vi "GetControlRefsFromVi.vi"(11 "VI Refnum":refnum<vi>) -> (0 "error out":errorcluster, 3 "Variant":variant)   [LabVIEW 2016, in "M1M3SupportEUI_Views.lvlib"]
uses:
  M1M3SupportEUI_Views.lvlib
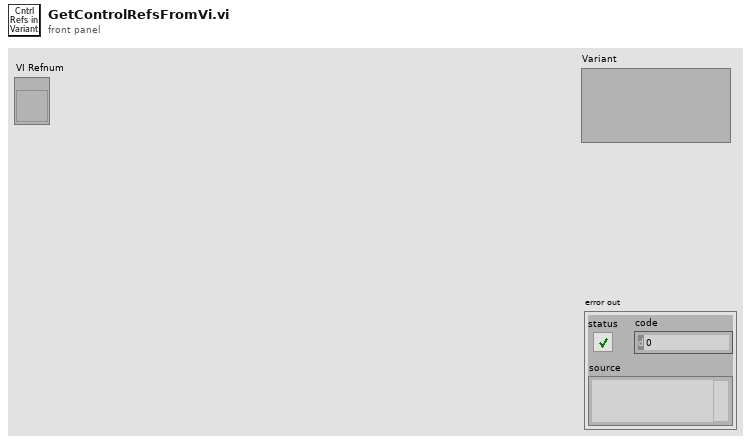
[diagram p1: front panel]
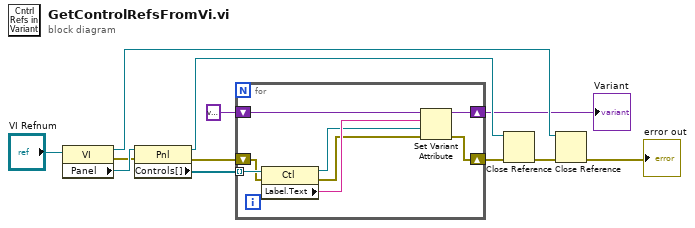
[diagram p0: block diagram]
diagram:
  n1 = property class="VI"(reference="VI Refnum") -> (reference out=w12:refnum<vi>, error out=w4:errorcluster, "Panel"=w5:refnum<vi>)  [unwired: 1 in]
  n2 = property class="Pnl"(reference=w5, error in=w4) -> (reference out=w11:refnum<vi>, error out=w8:errorcluster, "Controls[]"=w6:refnum<vi>[])
  n3 = for {
    tunnel: w6 -> [w20] mode=indexing
    shift-right: [w16] -> w2
    shift-left: variant -> [w19]
    shift-right: [w13] -> w10
    shift-left: w8 -> [w15]
    n4 = property class="Ctl"(reference=w20, error in=w15) -> (reference out=w17:refnum<vi>, error out=w14:errorcluster, "Label.Text"=w18:string)
    n5 = Set Variant Attribute(Variant=w19, name=w18, value=w17, error in=w14) -> (Variant out=w16:variant, error out=w13:errorcluster)  [unwired: 1 out]
  }
  "Variant" <- w2
  n6 = Close Reference(reference=w11, error in (no error)=w10) -> (error out=w9:errorcluster)
  n7 = Close Reference(reference=w12, error in (no error)=w9) -> (error out=→"error out":errorcluster)
